vi "Log Packet.vi"(4 "capture_usec":u32, 6 "capture_sec":u32, 8 "error in (no error)":errorcluster, 9 "capture_len":u32, 10 "capture_data_buffer":u8[](array[numeric]), 11 "pcap_dumper_reference":u64) -> (0 "error out":errorcluster, 3 "pcap_dumper_reference":u64)   [LabVIEW 2025, in "Automotive Ethernet Bus Monitor UI.lvlib" / "lvwpcap.lvlib"]
doc: "This VI writes an ethernet packet to a PCAP file dumper."
uses:
  lvwpcap.lvlib
  lvwpcap.dll
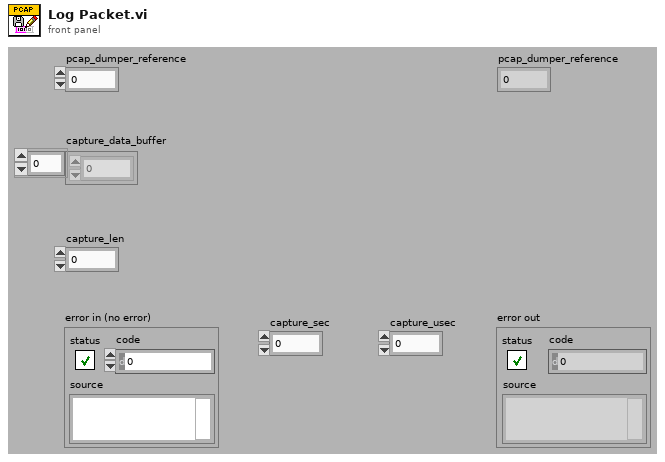
[diagram p1: front panel]
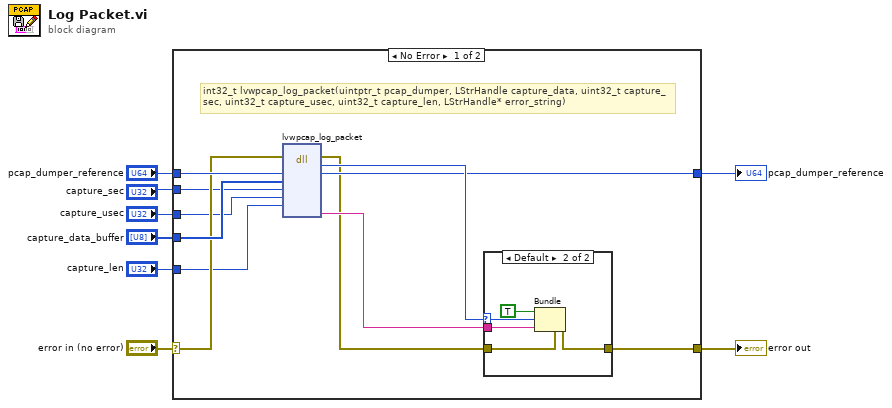
[diagram p0: block diagram]
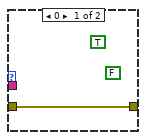
[diagram p2: hidden frame]
diagram:
  n1 = case shown="No Error" "error in (no error)" {
    selector: "error in (no error)" -> [w12 w27]
    tunnel: [w19 w27] -> w8
    tunnel: "pcap_dumper_reference" -> [w16 w26]
    tunnel: "capture_data_buffer" -> [w15 _]
    tunnel: [w14 w26] -> w4
    tunnel: "capture_sec" -> [w11 _]
    tunnel: "capture_usec" -> [w10 _]
    tunnel: "capture_len" -> [w9 _]
    frame No Error {
      # "int32_t lvwpcap_log_packet(uintptr_t pcap_dumper, LStrHandle capture_data, uint32_t capture_sec, uint32_t capture_usec, uint32_t capture_len, LStrHandle* error_string)"
      n2 = dll-call lib="lvwpcap.*" fn="lvwpcap_log_packet"(error in=w12, "pcap_dumper"=w16, "capture_data"=w15, "capture_sec"=w11, "capture_usec"=w10, "capture_len"=w9) -> (error out=w13:errorcluster, "return type"=w18:i32, "pcap_dumper"=w14:u64, "error_string"=w17:string)  [unwired: 7 in, 1 out]
      n3 = case shown="Default" w18 {
        selector: w18 -> [_ w24]
        tunnel: w17 -> [_ w23]
        tunnel: w13 -> [w20 w25]
        tunnel: [w20 w21] -> w19
        frame 0 {
          (unwired) FALSE
          (unwired) TRUE
        }
        frame Default {
          n4 = Bundle(cluster=w25, "status"=TRUE, "code"=w24, "source"=w23) -> (w21:errorcluster)
        }
      }
    }
    frame Error {
    }
  }
  "error out" <- w8
  "pcap_dumper_reference" <- w4
